vi "Write Single Register Response.vi"(8 "error in":errorcluster, 10 "modbus data unit in":refnum<class "Modbus Data Unit.lvclass">) -> (0 "error out":errorcluster, 1 "Number of Coils":u16, 2 "Address":u16)   [LabVIEW 2013, in "Modbus Library - Advance.lvlib" / "Master Function Definition.lvclass"]
doc: "Decodes the response for the write single register function."
uses:
  Master Function Definition.lvclass
  Modbus Data Unit/Modbus Data Unit.lvclass
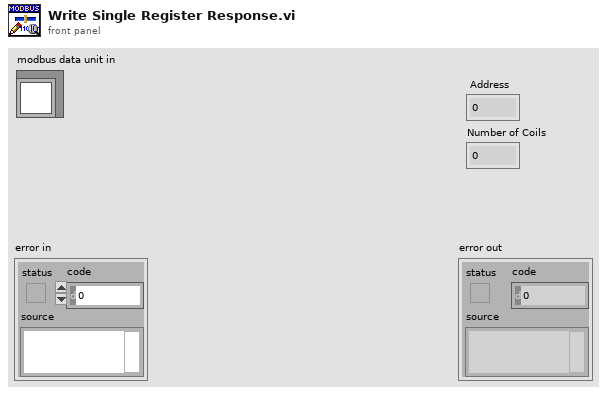
[diagram p1: front panel]
types:
  T1 = typedef "Modbus Library - Advance.lvlib/Modbus Data Unit.lvclass/Function.ctl" = u8
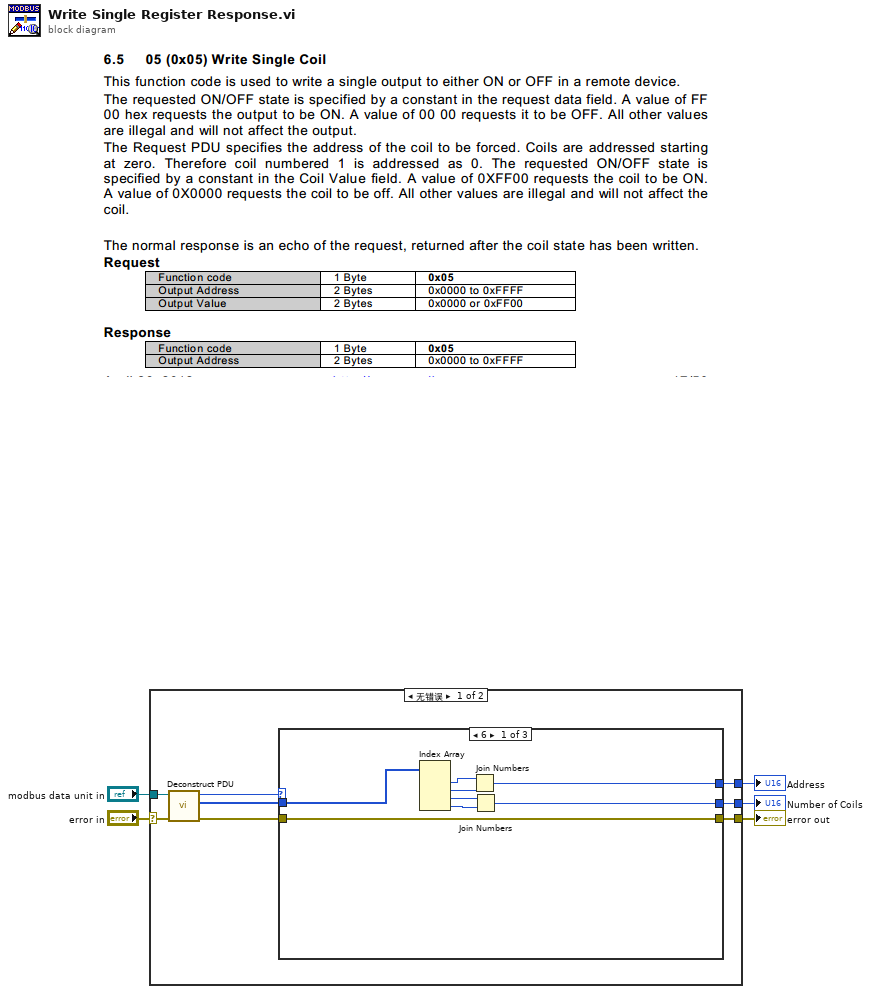
[diagram p0: block diagram]
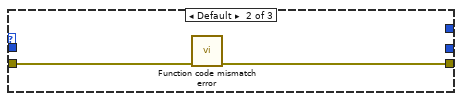
[diagram p2: hidden frame]
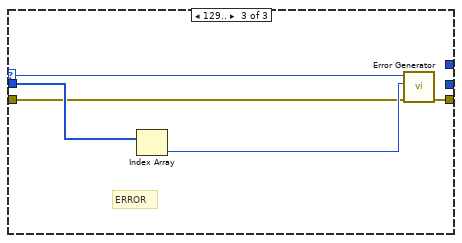
[diagram p3: hidden frame]
diagram:
  n1 = case shown="无错误" "error in" {
    selector: "error in" -> [w12 w29]
    tunnel: [w13 w29] -> w4
    tunnel: "modbus data unit in" -> [w10 _]
    tunnel: [w8 _] -> w2
    tunnel: [w7 _] -> w1
    frame No Error {
      n2 = call "Deconstruct PDU.vi"("error in"=w12, "modbus data unit in"=w10) -> ("error out"=w9:errorcluster, "data"=w11:u8[], "Function"=w6:T1)  [unwired: 7 in]
      n3 = case shown="6" w6 {
        selector: w6 -> [_ _ w24]
        tunnel: w9 -> [w20 w23 w25]
        tunnel: w11 -> [w21 _ w28]
        tunnel: [w20 w22 w27] -> w13
        tunnel: [w19 _ _] -> w8
        tunnel: [w18 _ _] -> w7
        frame 6 {
          n4 = Index Array(array=w21) -> (element #1=w17:u8, element #2=w16:u8, element #3=w15:u8, element #4=w14:u8)  [unwired: 4 in]
          n5 = Join Numbers(hi=w17, lo=w16) -> ((hi.lo)=w19:u16)
          n6 = Join Numbers(hi=w15, lo=w14) -> ((hi.lo)=w18:u16)
        }
        frame Default {
          n7 = call "Function code mismatch error.vi"("error in (no error)"=w23) -> ("error out"=w22:errorcluster)  [unwired: 10 in]
        }
        frame 129.. {
          # "ERROR"
          n8 = Index Array(array=w28) -> (element=w26:u8)  [unwired: 1 in]
          n9 = call "Error Generator.vi"("error in"=w25, "data return (error code)"=w26, "function return"=w24) -> ("error out"=w27:errorcluster)  [unwired: 8 in]
        }
      }
    }
    frame Error {
    }
  }
  "error out" <- w4
  "Address" <- w2
  "Number of Coils" <- w1
